vi "VersionCheck.vi"(0 "Version":string, 1 "error in (no error)":errorcluster) -> (2 "Latest Version":string, 3 "outdated?":bool, 4 "error out":errorcluster)   [LabVIEW 2020]
uses:
  <vilib>/regexp/Match Regular Expression.xnode
panel:
  out "standard output":string
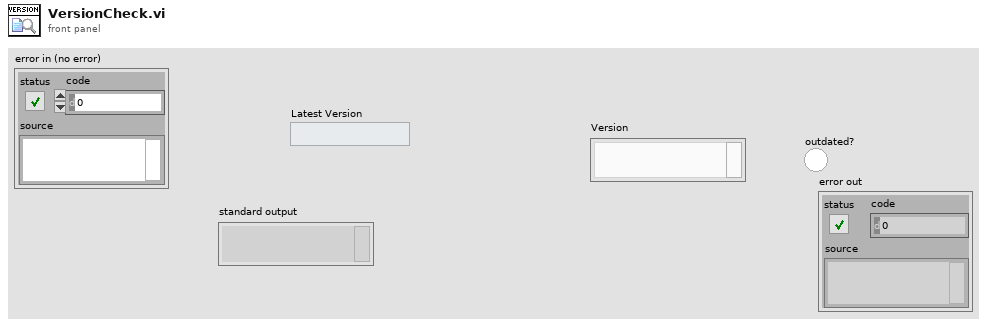
[diagram p1: front panel]
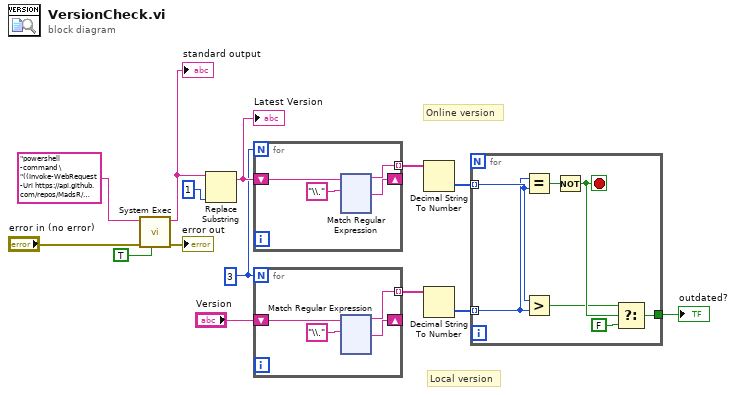
[diagram p0: block diagram]
diagram:
  w3 = 3
  # "Local version"
  # "Online version"
  n1 = call <vilib>:"System Exec.vi"("run minimized? (F)"=TRUE, "error in (no error)"="error in (no error)", "command line"="powershell -command \"((Invoke-WebRequest -Uri https://api.github.com/repos/MadsR/Ice-Nucleation/releases/latest).Content | ConvertFrom-Json).tag_name\"") -> ("error out"=→"error out":errorcluster, "standard output"=w12:string)  [unwired: 5 in, 2 out]
  "standard output" <- w12
  n2 = Replace Substring(2:1 ("length (len. of substring)"), 5:w12) -> (1:w10:string)  [unwired: 2 in, 1 out]
  "Latest Version" <- w10
  n3 = for {
    N: w3 -> [_]
    shift-right: [w16] -> _
    shift-left: w10 -> [w17]
    tunnel: [w15] -> w9 mode=indexing
    n4 = xnode "Match Regular Expression"("input string"=w17, "regular expression"="\\.") -> ("before match"=w15:string, "after match"=w16:string)  [unwired: 4 in, 3 out]
  }
  n5 = for {
    N: w3 -> [_]
    shift-right: [w134] -> _
    shift-left: "Version" -> [w135]
    tunnel: [w133] -> w7 mode=indexing
    n6 = xnode "Match Regular Expression"("input string"=w135, "regular expression"="\\.") -> ("before match"=w133:string, "after match"=w134:string)  [unwired: 4 in, 3 out]
  }
  n7 = Decimal String To Number(string=w9) -> (number=w8:i32[])  [unwired: 2 in, 1 out]
  n8 = Decimal String To Number(string=w7) -> (number=w5:i32[])  [unwired: 2 in, 1 out]
  n9 = for {
    tunnel: w8 -> [w256] mode=indexing
    tunnel: w5 -> [w255] mode=indexing
    tunnel: [w251] -> w4
    stop <- w254 stop-if-true
    n10 = Equal?(x=w255, y=w256) -> (x = y?=w257:bool)
    n11 = Greater?(x=w256, y=w255) -> (0:w253:bool)
    n12 = Not(x=w257) -> (.not. x?=w254:bool)
    n13 = Select(t=w253, s=w254, f=FALSE) -> (s? t:f=w251:bool)
  }
  "outdated?" <- w4
